vi "Count.vi"(8 "error in (no error)":errorcluster, 11 "StringList in":refnum<class "StringList.lvclass">) -> (0 "error out":errorcluster, 2 "Number of Items":i32, 3 "StringList out":refnum<class "StringList.lvclass">)   [LabVIEW 2013, in "LapDog.Collections.v_.Lists.lvlib" / "StringList.lvclass"]
uses:
  StringList.lvclass
  ObjectList/ObjectList.lvclass
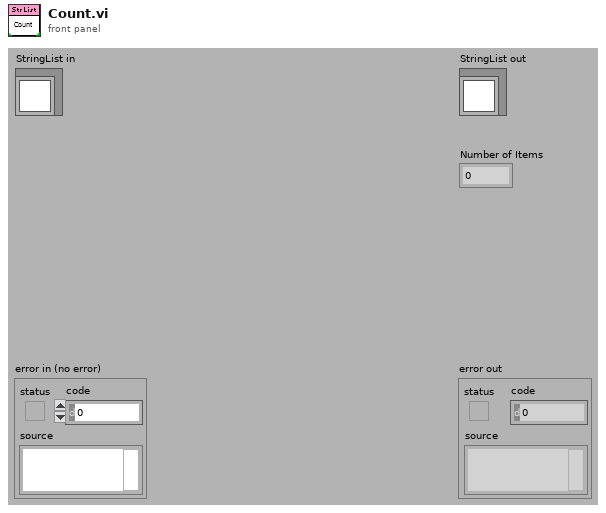
[diagram p1: front panel]
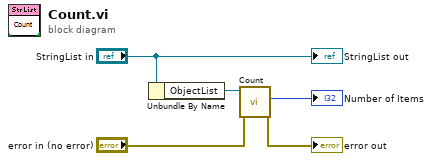
[diagram p0: block diagram]
diagram:
  n1 = Unbundle By Name("StringList in") -> ("ObjectList"=w4:refnum<class "ObjectList.lvclass">)
  n2 = call-dynamic "Count.vi"("error in (no error)"="error in (no error)", "List in"=w4) -> ("error out"=→"error out":errorcluster, "Number of Items"=→"Number of Items":i32)  [unwired: 7 in, 1 out]
  "StringList out" <- "StringList in"
